vi "判断单行.vi"(11 "数组":u32[](array[colorbox])) -> (2 "是否空行":bool, 3 "是否满行":bool)   [LabVIEW 2012]
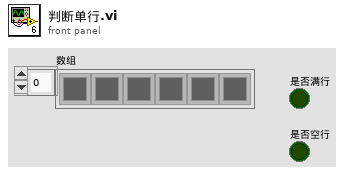
[diagram p1: front panel]
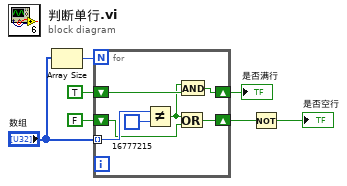
[diagram p0: block diagram]
diagram:
  n1 = Array Size(array="数组") -> (size(s)=w2:i32)
  n2 = for {
    N: w2 -> [_]
    tunnel: "数组" -> [w14] mode=indexing
    shift-right: [w11] -> w5
    shift-left: TRUE -> [w12]
    shift-right: [w8] -> w4
    shift-left: FALSE -> [w10]
    n3 = Not Equal?(x=w14, y=u32 16777215) -> (x != y?=w9:bool)
    n4 = Or(x=w9, y=w10) -> (x .or. y?=w8:bool)
    n5 = And(x=w9, y=w12) -> (x .and. y?=w11:bool)
  }
  "是否满行" <- w5
  n6 = Not(x=w4) -> (.not. x?=→"是否空行":bool)
